vi "Temperature Read Single.vi"(8 "error in":errorcluster, 9 "Channel Index":i32=1, 11 "Climate Chamber in":refnum<class "Climate Chamber.lvclass">) -> (0 "error out":errorcluster, 1 "Changed or First Call?":bool, 2 "Temperature SP":dbl, 3 "Climate Chamber out":refnum<class "Climate Chamber.lvclass">)   [LabVIEW 2023, in "Climate Chamber.lvclass"]
uses:
  Climate Chamber.lvclass
  Climate Chamber.lvclass/Climate Chamber.ctl
  Low Level Capabilities/Temperature/Temperature Setpoint/Temperature Setpoint.lvclass
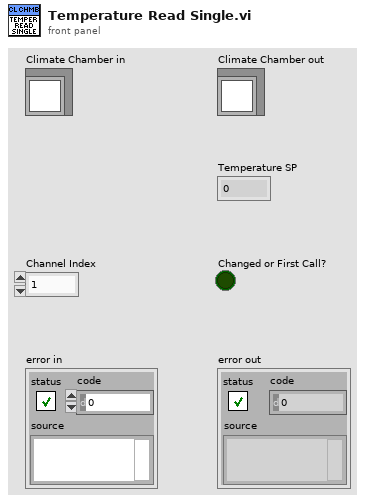
[diagram p1: front panel]
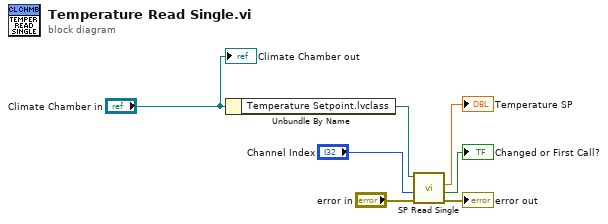
[diagram p0: block diagram]
diagram:
  n1 = Unbundle By Name("Climate Chamber in") -> ("Temperature Setpoint.lvclass"=w6:refnum<class "Temperature Setpoint.lvclass">)
  n2 = call-dynamic "SP Read Single.vi"("error in"="error in", "Channel Index"="Channel Index", "Temperature Setpoint in"=w6) -> ("error out"=→"error out":errorcluster, "Changed or First Call?"=→"Changed or First Call?":bool, "Temperature SP"=→"Temperature SP":dbl)  [unwired: 5 in, 1 out]
  "Climate Chamber out" <- "Climate Chamber in"
